vi "InclinometerSampleSensorLoop.vi"   [LabVIEW 2016]
uses:
  InclinometerSampleSensorLoopData.ctl
  InclinometerSampleSensorLoopStates.ctl
  InclinometerSample.ctl
  InclinometerErrorSample.ctl
  InclinometerErrorCodes.ctl
  <vilib>/Platform/TimedLoop/XDataNode/timing_clust.ctl
  <vilib>/Platform/TimedLoop/XDataNode/nitl_modes.ctl
  <vilib>/Platform/TimedLoop/XDataNode/wakeup.ctl
  <vilib>/rvi/Emulation/niFpgaSctlEmulationGetInTimedLoop.vi
  <vilib>/rvi/Emulation/niFpgaEmulationReportErrorSimple.vi
  <vilib>/rvi/Emulation/niFpgaGetClockAttributes.vi
  <vilib>/rvi/Emulation/niFpgaCriticalErrorInLSC.vi
  <vilib>/rvi/Emulation/niFpgaEmulationIsFPGAContextNoSignature.vi
  <vilib>/rvi/errors/niFpgaSetErrorForExecOnDevCompSimple.vi
  <vilib>/rvi/eio/common/nirviEmuReportErrorAndStop.vi
  <vilib>/rvi/DataTransferAndStorage/Container/Common/niFpgaContainerGetUniqueNameForEmu.vi
  <vilib>/rvi/FIFO/Fifo_Resource/nirvififoEmulationSetSize.vi
  <vilib>/rvi/FIFO/Fifo_Resource/nirviFifoEmulationQueueMgr.vi
  <instcachedir>/0/nirviFifoEmulationQueueMgr_E5CAEC123FF24DC58D834DCA3CDAA9B5.lvgen/nirviFifoEmulationQueueMgr_E5CAEC123FF24DC58D834DCA3CDAA9B5_004.vi
  <vilib>/Utility/error.llb/Clear Errors.vi
  <vilib>/rvi/FIFO/Fifo_Resource/nirvififoEmulationCreateLock.vi
  <vilib>/rvi/Emulation/niFpgaProcessEmulError.vi
  <vilib>/rvi/FIFO/Fifo_Resource/nirvififoEmulationObtainLock.vi
  <vilib>/rvi/FIFO/Fifo_Resource/nirvififoEmulationReleaseLock.vi
  <vilib>/rvi/occurrence/nirviWaitOnOccurrenceBase.vi
  <vilib>/rvi/errors/nirviReportUnexpectedCaseInternalError.vi
  <vilib>/rvi/errors/nirviReportUnexpectedCaseInternalError (U32).vi
  <vilib>/rvi/FIFO/Fifo_Resource/nirvififoEmulationDetermineInputValidOut.vi
  <instcachedir>/0/nirviFifoEmulationQueueMgr_E5CAEC123FF24DC58D834DCA3CDAA9B5.lvgen/nirviFifoEmulationQueueMgr_E5CAEC123FF24DC58D834DCA3CDAA9B5_009.vi
  <instcachedir>/0/nirviFifoEmulationQueueMgr_E5CAEC123FF24DC58D834DCA3CDAA9B5.lvgen/nirviFifoEmulationQueueMgr_E5CAEC123FF24DC58D834DCA3CDAA9B5_002.vi
  <vilib>/rvi/Memory/Memory_Emulation/niFpgaMemoryEmulationCacheClearOnFirstRun.vi
  <vilib>/rvi/Memory/Memory_Emulation/nirvimemoryEmulationManagerCache_MakeExclusive.vi
  <vilib>/rvi/Memory/Memory_Emulation/niFpgaMemoryEmulationValidateCache.vi
  <vilib>/rvi/Memory/Memory_Emulation/nirvimemoryEmulationManagerCache_InsertValue.vi
  <vilib>/rvi/Memory/Memory_Emulation/nirvimemoryEmulationManagerCache_ReleaseExclusive.vi
  <vilib>/rvi/Memory/Memory_Emulation/nirvimemoryEmulationManagerCache_GetValue.vi
  <vilib>/rvi/Memory/Memory_Emulation/nirvimemoryEmulationManagerCache_SetValue.vi
  <instcachedir>/0/nirviFifoEmulationQueueMgr_E5CAEC123FF24DC58D834DCA3CDAA9B5.lvgen/nirviFifoEmulationQueueMgr_E5CAEC123FF24DC58D834DCA3CDAA9B5_046.vi
  <instcachedir>/0/nirviFifoEmulationQueueMgr_E5CAEC123FF24DC58D834DCA3CDAA9B5.lvgen/nirviFifoEmulationQueueMgr_E5CAEC123FF24DC58D834DCA3CDAA9B5_033.vi
  <vilib>/Platform/TimedLoop/XDataNode/XDataNode.xnode
  <vilib>/rvi/DataTransferAndStorage/Container/XNode/niFpgaContainer.xnode
  <vilib>/rvi/FIFO/Fifo_Resource/nirvififoEmulationRead.vi
  <vilib>/rvi/FIFO/Fifo_Resource/nirvififoEmulationWrite.vi
  <vilib>/rvi/DataTransferAndStorage/Register/Emulation/niFpgaRegisterEmulation.vi
  <vilib>/Platform/TimedLoop/XDataNode/XDNodeRunTimeDep.lvlib
types:
  T1 = typedef "InclinometerSampleSensorLoopData.ctl" = cluster{"State":T2, "Timestamp":u64, "Timeout":i32, "Angle":u32, "CRC":u16, "Exception":u8, "Sample":T3, "ErrorSample":T4}
  T2 = typedef "InclinometerSampleSensorLoopStates.ctl" = enum16{"WaitForTrigger", "ClearRxFIFO", "WaitForClearComplete", "WriteAddress", "WriteFunction", "WriteStartAddress1", "WriteStartAddress0", "WriteAddressCount1", "WriteAddressCount0", "WriteCRC1", "WriteCRC0", "ReadAddress", "ReadFunction", "ReadByteCount", "ReadDataByte1", "ReadDataByte0", "ReadDataByte3", "ReadDataByte2", "ReadCRCByte0", "ReadCRCByte1", "CalculateCRC", "ValidateCRC", "PrepareSample", "MoveSample", "ReadExceptionCode", "ReadExceptionCRCByte0", "ReadExceptionCRCByte1", "CalculateExceptionCRC", "ValidateExceptionCRC", "ParseExceptionCode", "ResponseAddressError", "ResponseFunctionCodeError", "ResponseByteCountError", "ResponseCRCError", "ResponseUnknownError", "ResponseTimeoutError", "SensorReportsIllegalFunction", "SensorReportsIllegalDataAddress", "PrepareErrorCode", "MoveErrorCode"}
  T3 = typedef "InclinometerSample.ctl" = cluster{"Timestamp":u64, "TxBytes":u64, "RxBytes":u64, "TxFrames":u64, "RxFrames":u64, "RawAngle":i32}
  T4 = typedef "InclinometerErrorSample.ctl" = cluster{"Timestamp":u64, "TxBytes":u64, "RxBytes":u64, "TxFrames":u64, "RxFrames":u64, "ErrorCode":T5}
  T5 = typedef "InclinometerErrorCodes.ctl" = enum8{"None", "ResponseAddressError", "ResponseFunctionCodeError", "ResponseByteCountError", "ResponseCRCError", "ResponseUnknownError", "ResponseTimeoutError", "SensorReportsIllegalFunction", "SensorReportsIllegalDataAddress"}
  T6 = typedef "XDNodeRunTimeDep.lvlib/timing_clust.ctl" = cluster{"Expected End [f-1]":u64, "Actual End [f-1]":u64, "Finished Late? [f-1]":bool, "Expected End [i-1]":u64, "Actual End [i-1]":u64, "Finished Late? [i-1]":bool, "Expected Start [i]":u64, "Actual Start [i]":u64, "Expected Start [f]":u64, "Actual Start [f]":u64, "Source Name":string, "Structure Name":string, "Period":i64, "Deadline":i64, "Offset":i64, "Start":i64, "Priority":i32, "Timeout":i32, "Mode":T7, "Wakeup Reason":T8, "Error":errorcluster, "Source Type":string, "Secondary Source Type":string, "Global End Time":u64, "Global Start Time":u64, "Frame Duration":u64, "Iteration Duration":u64, "Assigned CPU":i32, "I/O Scan Engine Mode":u32}
  T7 = typedef "XDNodeRunTimeDep.lvlib/nitl_modes.ctl" = enum32{"No Change", "Process missed periods, maintain original phase", "Discard missed periods, maintain original phase", "Process missed periods, ignore original phase", "Discard missed periods, ignore original phase"}
  T8 = typedef "XDNodeRunTimeDep.lvlib/wakeup.ctl" = enum32{"Normal", "Aborted", "Asynchronous wakeup", "Timing source error", "Timed loop error", "Timeout"}
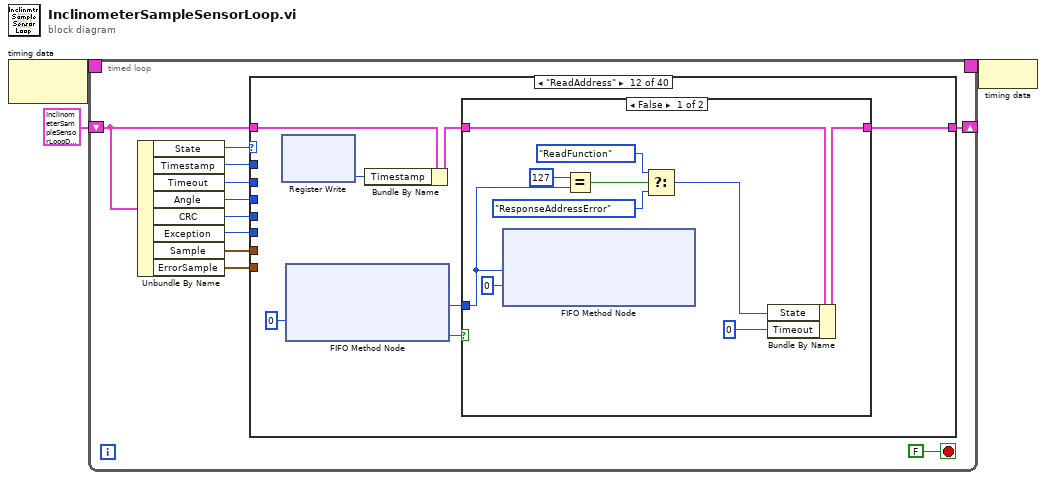
[diagram p0: block diagram]
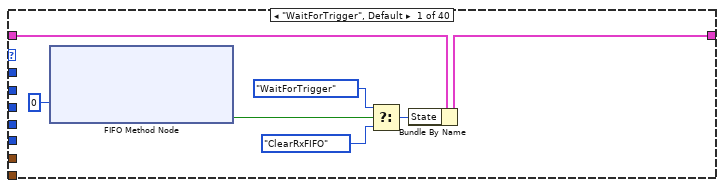
[diagram p2: hidden frame]
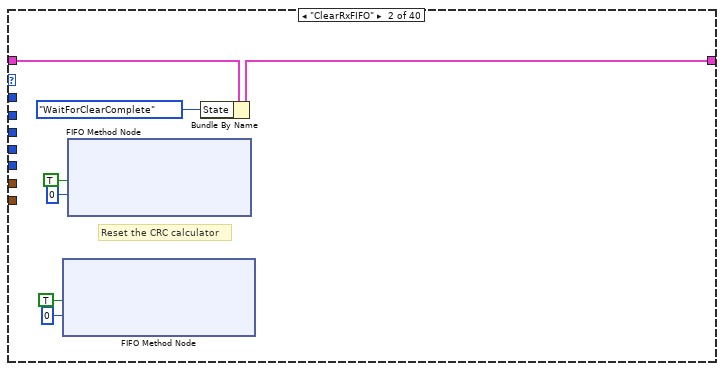
[diagram p3: hidden frame]
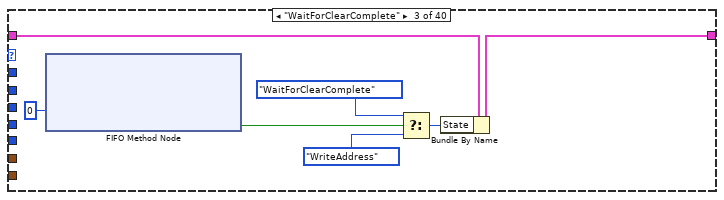
[diagram p4: hidden frame]
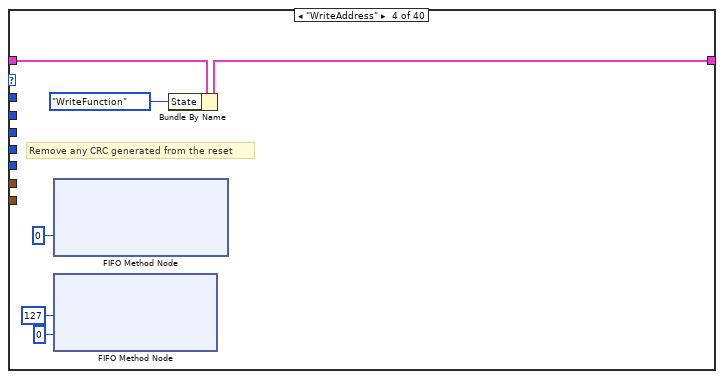
[diagram p5: hidden frame]
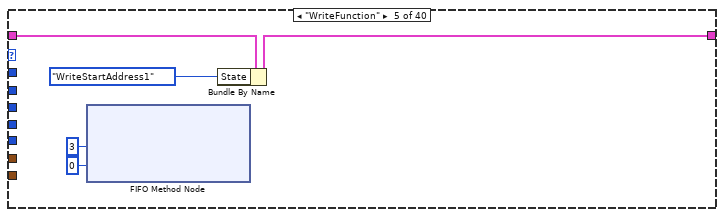
[diagram p6: hidden frame]
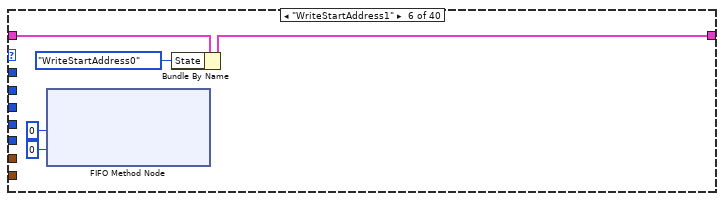
[diagram p7: hidden frame]
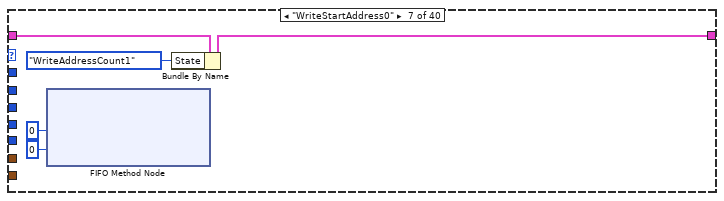
[diagram p8: hidden frame]
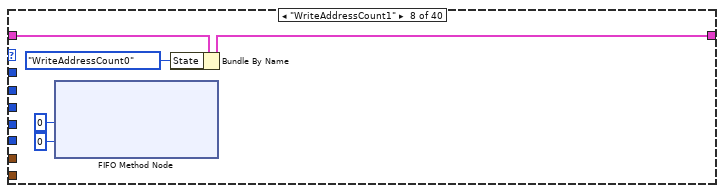
[diagram p9: hidden frame]
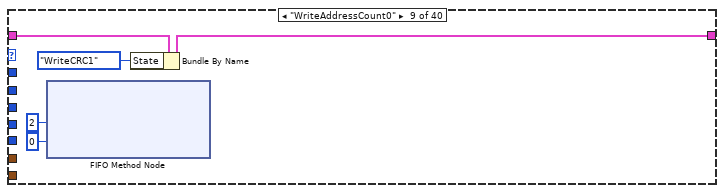
[diagram p10: hidden frame]
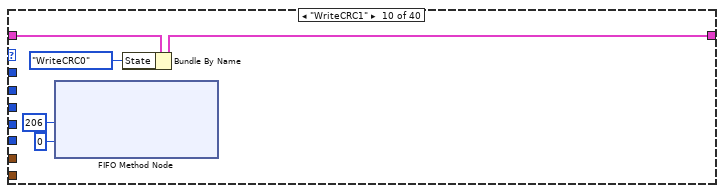
[diagram p11: hidden frame]
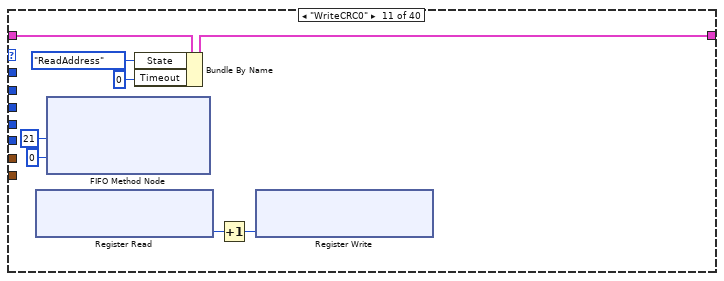
[diagram p12: hidden frame]
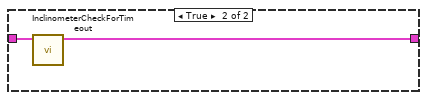
[diagram p13: hidden frame]
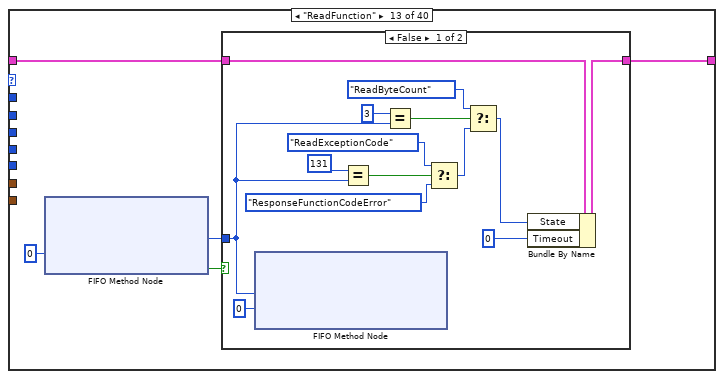
[diagram p14: hidden frame]
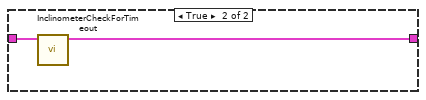
[diagram p15: hidden frame]
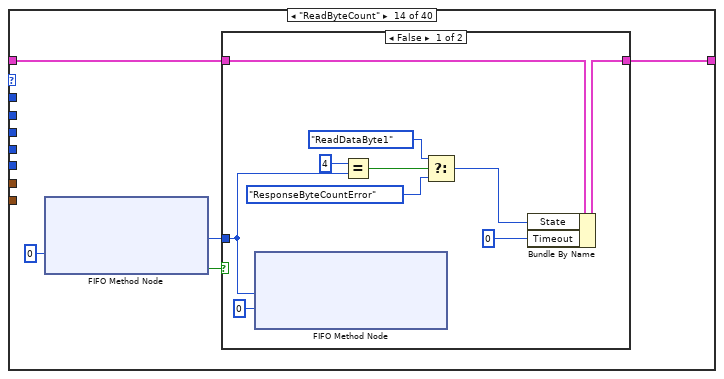
[diagram p16: hidden frame]
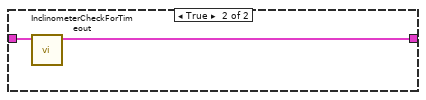
[diagram p17: hidden frame]
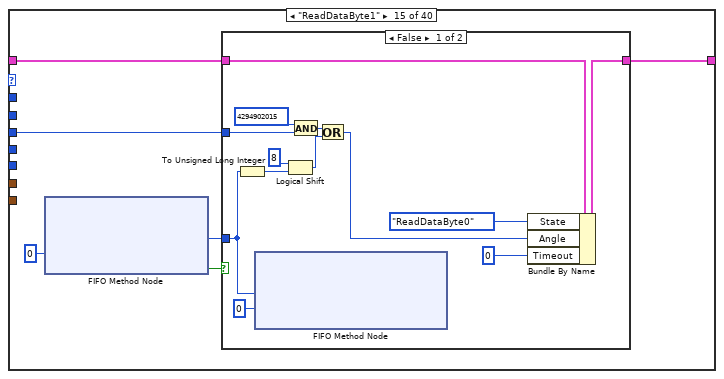
[diagram p18: hidden frame]
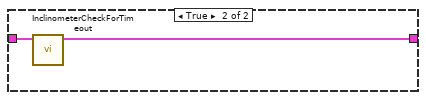
[diagram p19: hidden frame]
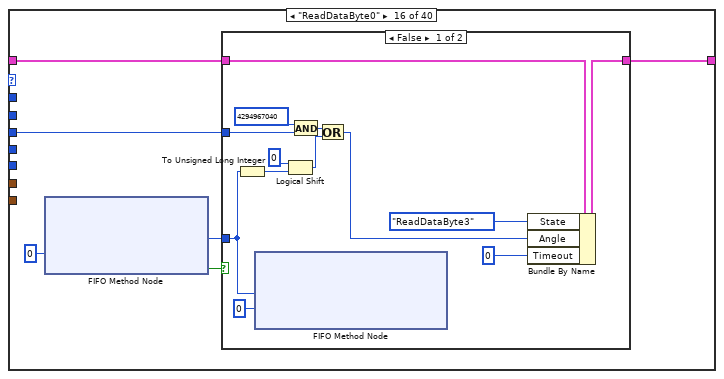
[diagram p20: hidden frame]
diagram:
  n1 = node-c288() -> (w3:T6)  [unwired: 1 in]
  n2 = timed-loop {
    timing: w3 -> [_]
    timing-out: [_] -> w2
    shift-right: [w13] -> _
    shift-left: T1 {"State"=enum."WaitForTrigger", "Timestamp"=0, "Timeout"=0, "Angle"=0, "CRC"=0, "Exception"=0, "Sample"={"Timestamp"=0, "TxBytes"=0, "RxBytes"=0, "TxFrames"=0, "RxFrames"=0, "RawAngle"=0}, "ErrorSample"={"Timestamp"=0, "TxBytes"=0, "RxBytes"=0, "TxFrames"=0, "RxFrames"=0, "ErrorCode"=enum."None"}} ("InclinometerData") -> [w14]
    stop <- FALSE stop-if-true
    n3 = Unbundle By Name(w14) -> ("State"=w12:T2, "Timestamp"=w7:u64, "Timeout"=w11:i32, "Angle"=w10:u32, "CRC"=w9:u16, "Exception"=w6:u8, "Sample"=w5:T3, "ErrorSample"=w4:T4)
    n4 = case shown="\"ReadAddress\"" w12 {
      tunnel: w14 -> [w20 w27 w34 w40 w45 w50 w55 w60 w65 w70 w78 w82 w99 w120 w138 w159 w180 w201 w222 w242 w264 w267 w290 w295 w297 w318 w338 w360 w363 w385 w389 w393 w397 w401 w405 w409 w413 w417 w425 w430]
      tunnel: [w21 w28 w35 w41 w46 w51 w56 w61 w66 w71 w79 w83 w100 w121 w139 w160 w181 w202 w223 w243 w265 w268 w291 w296 w298 w319 w339 w361 w364 w386 w390 w394 w398 w402 w406 w410 w414 w418 w426 w431] -> w13
      tunnel: w11 -> [_ _ _ _ _ _ _ _ _ _ _ _ _ _ _ _ _ _ _ _ _ _ _ _ _ _ _ _ _ _ _ _ _ _ _ _ _ _ _ _]
      tunnel: w10 -> [_ _ _ _ _ _ _ _ _ _ _ _ _ _ w137 w158 w179 w200 _ _ _ _ w284 _ _ _ _ _ _ _ _ _ _ _ _ _ _ _ _ _]
      tunnel: w9 -> [_ _ _ _ _ _ _ _ _ _ _ _ _ _ _ _ _ _ w221 w241 _ w266 _ _ _ w317 w337 _ w362 _ _ _ _ _ _ _ _ _ _ _]
      tunnel: w7 -> [_ _ _ _ _ _ _ _ _ _ _ _ _ _ _ _ _ _ _ _ _ _ w289 _ _ _ _ _ _ _ _ _ _ _ _ _ _ _ w424 _]
      tunnel: w6 -> [_ _ _ _ _ _ _ _ _ _ _ _ _ _ _ _ _ _ _ _ _ _ _ _ _ _ _ _ _ w380 _ _ _ _ _ _ _ _ _ _]
      tunnel: w5 -> [_ _ _ _ _ _ _ _ _ _ _ _ _ _ _ _ _ _ _ _ _ _ _ w294 _ _ _ _ _ _ _ _ _ _ _ _ _ _ _ _]
      tunnel: w4 -> [_ _ _ _ _ _ _ _ _ _ _ _ _ _ _ _ _ _ _ _ _ _ _ _ _ _ _ _ _ _ _ _ _ _ _ _ _ _ _ w427]
      frame "WaitForTrigger", Default {
        n5 = xnode ("FIFO Method Node")("Timeout"=0) -> ("Timed Out?"=w15:bool)  [unwired: 1 in, 2 out]
        n6 = Select(t=InclinometerSampleSensorLoopStates."WaitForTrigger" ("InclinometerState"), s=w15, f=InclinometerSampleSensorLoopStates."ClearRxFIFO" ("InclinometerState")) -> (s? t:f=w17:T2)
        n7 = Bundle By Name(cluster=w20, "State"=w17) -> (w21:T1)
      }
      frame "ClearRxFIFO" {
        # "Reset the CRC calculator"
        n8 = xnode ("FIFO Method Node")("Element"=TRUE, "Timeout"=0) -> ()  [unwired: 1 in, 2 out]
        n9 = xnode ("FIFO Method Node")("Element"=TRUE, "Timeout"=0) -> ()  [unwired: 1 in, 2 out]
        n10 = Bundle By Name(cluster=w27, "State"=InclinometerSampleSensorLoopStates."WaitForClearComplete" ("InclinometerState")) -> (w28:T1)
      }
      frame "WaitForClearComplete" {
        n11 = xnode ("FIFO Method Node")("Timeout"=0) -> ("Timed Out?"=w29:bool)  [unwired: 1 in, 2 out]
        n12 = Select(t=InclinometerSampleSensorLoopStates."WaitForClearComplete", s=w29, f=InclinometerSampleSensorLoopStates."WriteAddress" ("InclinometerState")) -> (s? t:f=w31:T2)
        n13 = Bundle By Name(cluster=w34, "State"=w31) -> (w35:T1)
      }
      frame "WriteAddress" {
        # "Remove any CRC generated from the reset"
        n14 = xnode ("FIFO Method Node")("Timeout"=0) -> ()  [unwired: 1 in, 3 out]
        n15 = xnode ("FIFO Method Node")("Element"=u8 127, "Timeout"=0) -> ()  [unwired: 1 in, 2 out]
        n16 = Bundle By Name(cluster=w40, "State"=InclinometerSampleSensorLoopStates."WriteFunction" ("InclinometerState")) -> (w41:T1)
      }
      frame "WriteFunction" {
        n17 = xnode ("FIFO Method Node")("Element"=u8 3, "Timeout"=0) -> ()  [unwired: 1 in, 2 out]
        n18 = Bundle By Name(cluster=w45, "State"=InclinometerSampleSensorLoopStates."WriteStartAddress1" ("InclinometerState")) -> (w46:T1)
      }
      frame "WriteStartAddress1" {
        n19 = xnode ("FIFO Method Node")("Element"=u8 0, "Timeout"=0) -> ()  [unwired: 1 in, 2 out]
        n20 = Bundle By Name(cluster=w50, "State"=InclinometerSampleSensorLoopStates."WriteStartAddress0" ("InclinometerState")) -> (w51:T1)
      }
      frame "WriteStartAddress0" {
        n21 = xnode ("FIFO Method Node")("Element"=u8 0, "Timeout"=0) -> ()  [unwired: 1 in, 2 out]
        n22 = Bundle By Name(cluster=w55, "State"=InclinometerSampleSensorLoopStates."WriteAddressCount1" ("InclinometerState")) -> (w56:T1)
      }
      frame "WriteAddressCount1" {
        n23 = xnode ("FIFO Method Node")("Element"=u8 0, "Timeout"=0) -> ()  [unwired: 1 in, 2 out]
        n24 = Bundle By Name(cluster=w60, "State"=InclinometerSampleSensorLoopStates."WriteAddressCount0" ("InclinometerState")) -> (w61:T1)
      }
      frame "WriteAddressCount0" {
        n25 = xnode ("FIFO Method Node")("Element"=u8 2, "Timeout"=0) -> ()  [unwired: 1 in, 2 out]
        n26 = Bundle By Name(cluster=w65, "State"=InclinometerSampleSensorLoopStates."WriteCRC1" ("InclinometerState")) -> (w66:T1)
      }
      frame "WriteCRC1" {
        n27 = xnode ("FIFO Method Node")("Element"=u8 206, "Timeout"=0) -> ()  [unwired: 1 in, 2 out]
        n28 = Bundle By Name(cluster=w70, "State"=InclinometerSampleSensorLoopStates."WriteCRC0" ("InclinometerState")) -> (w71:T1)
      }
      frame "WriteCRC0" {
        n29 = xnode ("Register Read")() -> ("Data"=w73:u64)  [unwired: 1 in, 1 out]
        n30 = xnode ("FIFO Method Node")("Element"=u8 21, "Timeout"=0) -> ()  [unwired: 1 in, 2 out]
        n31 = Bundle By Name(cluster=w78, "State"=InclinometerSampleSensorLoopStates."ReadAddress" ("InclinometerState"), "Timeout"=0) -> (w79:T1)
        n32 = Increment(x=w73) -> (x+1=w72:u64)
        n33 = xnode ("Register Write")("Data"=w72) -> ()  [unwired: 1 in, 1 out]
      }
      frame "ReadAddress" {
        n34 = xnode "Register Write"() -> ("Data"=w80:u64)  [unwired: 1 in, 1 out]
        n35 = xnode ("FIFO Method Node")("Timeout"=0) -> ("Element"=w84:u8, "Timed Out?"=w85:bool)  [unwired: 1 in, 1 out]
        n36 = Bundle By Name(cluster=w82, "Timestamp"=w80) -> (w81:T1)
        n37 = case shown="False" w85 {
          tunnel: w84 -> [w93 _]
          tunnel: [w95 w97] -> w83
          tunnel: w81 -> [w96 w98]
          frame False {
            n38 = xnode ("FIFO Method Node")("Element"=w93, "Timeout"=0) -> ()  [unwired: 1 in, 2 out]
            n39 = Equal?(x=u8 127, y=w93) -> (x = y?=w91:bool)
            n40 = Select(t=InclinometerSampleSensorLoopStates."ReadFunction" ("InclinometerState"), s=w91, f=InclinometerSampleSensorLoopStates."ResponseAddressError" ("InclinometerState")) -> (s? t:f=w88:T2)
            n41 = Bundle By Name(cluster=w96, "State"=w88, "Timeout"=0) -> (w95:T1)
          }
          frame True {
            n42 = call "InclinometerCheckForTimeout.vi"("InclinometerSampleSensorLoopData in"=w98) -> ("InclinometerSampleSensorLoopData out"=w97:T1)  [unwired: 10 in]
          }
        }
      }
      frame "ReadFunction" {
        n43 = xnode ("FIFO Method Node")("Timeout"=0) -> ("Element"=w101:u8, "Timed Out?"=w102:bool)  [unwired: 1 in, 1 out]
        n44 = case shown="False" w102 {
          tunnel: w101 -> [w109 _]
          tunnel: [w116 w118] -> w100
          tunnel: w99 -> [w117 w119]
          frame False {
            n45 = xnode ("FIFO Method Node")("Element"=w109, "Timeout"=0) -> ()  [unwired: 1 in, 2 out]
            n46 = Equal?(x=u8 131, y=w109) -> (x = y?=w108:bool)
            n47 = Equal?(x=u8 3, y=w109) -> (x = y?=w113:bool)
            n48 = Select(t=InclinometerSampleSensorLoopStates."ReadExceptionCode" ("InclinometerState"), s=w108, f=InclinometerSampleSensorLoopStates."ResponseFunctionCodeError" ("InclinometerState")) -> (s? t:f=w111:T2)
            n49 = Select(t=InclinometerSampleSensorLoopStates."ReadByteCount" ("InclinometerState"), s=w113, f=w111) -> (s? t:f=w105:T2)
            n50 = Bundle By Name(cluster=w117, "State"=w105, "Timeout"=0) -> (w116:T1)
          }
          frame True {
            n51 = call "InclinometerCheckForTimeout.vi"("InclinometerSampleSensorLoopData in"=w119) -> ("InclinometerSampleSensorLoopData out"=w118:T1)  [unwired: 10 in]
          }
        }
      }
      frame "ReadByteCount" {
        n52 = xnode ("FIFO Method Node")("Timeout"=0) -> ("Element"=w122:u8, "Timed Out?"=w123:bool)  [unwired: 1 in, 1 out]
        n53 = case shown="False" w123 {
          tunnel: w122 -> [w131 _]
          tunnel: [w133 w135] -> w121
          tunnel: w120 -> [w134 w136]
          frame False {
            n54 = xnode ("FIFO Method Node")("Element"=w131, "Timeout"=0) -> ()  [unwired: 1 in, 2 out]
            n55 = Equal?(x=u8 4, y=w131) -> (x = y?=w129:bool)
            n56 = Select(t=InclinometerSampleSensorLoopStates."ReadDataByte1" ("InclinometerState"), s=w129, f=InclinometerSampleSensorLoopStates."ResponseByteCountError" ("InclinometerState")) -> (s? t:f=w126:T2)
            n57 = Bundle By Name(cluster=w134, "State"=w126, "Timeout"=0) -> (w133:T1)
          }
          frame True {
            n58 = call "InclinometerCheckForTimeout.vi"("InclinometerSampleSensorLoopData in"=w136) -> ("InclinometerSampleSensorLoopData out"=w135:T1)  [unwired: 10 in]
          }
        }
      }
      frame "ReadDataByte1" {
        n59 = xnode ("FIFO Method Node")("Timeout"=0) -> ("Element"=w140:u8, "Timed Out?"=w141:bool)  [unwired: 1 in, 1 out]
        n60 = case shown="False" w141 {
          tunnel: w140 -> [w146 _]
          tunnel: [w154 w156] -> w139
          tunnel: w138 -> [w155 w157]
          tunnel: w137 -> [w150 _]
          frame False {
            n61 = To Unsigned Long Integer(number=w146) -> (unsigned 32bit integer=w145:u32)
            n62 = xnode ("FIFO Method Node")("Element"=w146, "Timeout"=0) -> ()  [unwired: 1 in, 2 out]
            n63 = Logical Shift(y=i16 8, x=w145) -> (x << y=w148:u32)
            n64 = And(x=u32 4294902015, y=w150) -> (x .and. y?=w147:u32)
            n65 = Or(x=w147, y=w148) -> (x .or. y?=w144:u32)
            n66 = Bundle By Name(cluster=w155, "State"=InclinometerSampleSensorLoopStates."ReadDataByte0" ("InclinometerState"), "Angle"=w144, "Timeout"=0) -> (w154:T1)
          }
          frame True {
            n67 = call "InclinometerCheckForTimeout.vi"("InclinometerSampleSensorLoopData in"=w157) -> ("InclinometerSampleSensorLoopData out"=w156:T1)  [unwired: 10 in]
          }
        }
      }
      frame "ReadDataByte0" {
        n68 = xnode ("FIFO Method Node")("Timeout"=0) -> ("Element"=w161:u8, "Timed Out?"=w162:bool)  [unwired: 1 in, 1 out]
        n69 = case shown="False" w162 {
          tunnel: w161 -> [w167 _]
          tunnel: [w175 w177] -> w160
          tunnel: w159 -> [w176 w178]
          tunnel: w158 -> [w171 _]
          frame False {
            n70 = To Unsigned Long Integer(number=w167) -> (unsigned 32bit integer=w166:u32)
            n71 = xnode ("FIFO Method Node")("Element"=w167, "Timeout"=0) -> ()  [unwired: 1 in, 2 out]
            n72 = Logical Shift(y=i16 0, x=w166) -> (x << y=w169:u32)
            n73 = And(x=u32 4294967040, y=w171) -> (x .and. y?=w168:u32)
            n74 = Or(x=w168, y=w169) -> (x .or. y?=w165:u32)
            n75 = Bundle By Name(cluster=w176, "State"=InclinometerSampleSensorLoopStates."ReadDataByte3" ("InclinometerState"), "Angle"=w165, "Timeout"=0) -> (w175:T1)
          }
          frame True {
            n76 = call "InclinometerCheckForTimeout.vi"("InclinometerSampleSensorLoopData in"=w178) -> ("InclinometerSampleSensorLoopData out"=w177:T1)  [unwired: 10 in]
          }
        }
      }
      frame "ReadDataByte3" {
        n77 = xnode ("FIFO Method Node")("Timeout"=0) -> ("Element"=w182:u8, "Timed Out?"=w183:bool)  [unwired: 1 in, 1 out]
        n78 = case shown="False" w183 {
          tunnel: w182 -> [w188 _]
          tunnel: [w196 w198] -> w181
          tunnel: w180 -> [w197 w199]
          tunnel: w179 -> [w192 _]
          frame False {
            n79 = To Unsigned Long Integer(number=w188) -> (unsigned 32bit integer=w187:u32)
            n80 = xnode ("FIFO Method Node")("Element"=w188, "Timeout"=0) -> ()  [unwired: 1 in, 2 out]
            n81 = Logical Shift(y=i16 24, x=w187) -> (x << y=w190:u32)
            n82 = And(x=u32 16777215, y=w192) -> (x .and. y?=w189:u32)
            n83 = Or(x=w189, y=w190) -> (x .or. y?=w186:u32)
            n84 = Bundle By Name(cluster=w197, "State"=InclinometerSampleSensorLoopStates."ReadDataByte2" ("InclinometerState"), "Angle"=w186, "Timeout"=0) -> (w196:T1)
          }
          frame True {
            n85 = call "InclinometerCheckForTimeout.vi"("InclinometerSampleSensorLoopData in"=w199) -> ("InclinometerSampleSensorLoopData out"=w198:T1)  [unwired: 10 in]
          }
        }
      }
      frame "ReadDataByte2" {
        n86 = xnode ("FIFO Method Node")("Timeout"=0) -> ("Element"=w203:u8, "Timed Out?"=w204:bool)  [unwired: 1 in, 1 out]
        n87 = case shown="False" w204 {
          tunnel: w203 -> [w209 _]
          tunnel: [w217 w219] -> w202
          tunnel: w201 -> [w218 w220]
          tunnel: w200 -> [w213 _]
          frame False {
            n88 = To Unsigned Long Integer(number=w209) -> (unsigned 32bit integer=w208:u32)
            n89 = xnode ("FIFO Method Node")("Element"=w209, "Timeout"=0) -> ()  [unwired: 1 in, 2 out]
            n90 = Logical Shift(y=i16 16, x=w208) -> (x << y=w211:u32)
            n91 = And(x=u32 4278255615, y=w213) -> (x .and. y?=w210:u32)
            n92 = Or(x=w210, y=w211) -> (x .or. y?=w207:u32)
            n93 = Bundle By Name(cluster=w218, "State"=InclinometerSampleSensorLoopStates."ReadCRCByte0" ("InclinometerState"), "Angle"=w207, "Timeout"=0) -> (w217:T1)
          }
          frame True {
            n94 = call "InclinometerCheckForTimeout.vi"("InclinometerSampleSensorLoopData in"=w220) -> ("InclinometerSampleSensorLoopData out"=w219:T1)  [unwired: 10 in]
          }
        }
      }
      frame "ReadCRCByte0" {
        n95 = xnode ("FIFO Method Node")("Timeout"=0) -> ("Element"=w224:u8, "Timed Out?"=w225:bool)  [unwired: 1 in, 1 out]
        n96 = case shown="False" w225 {
          tunnel: w224 -> [w231 _]
          tunnel: [w237 w239] -> w223
          tunnel: w222 -> [w238 w240]
          tunnel: w221 -> [w228 _]
          frame False {
            n97 = To Unsigned Word Integer(number=w231) -> (unsigned 16bit integer=w230:u16)
            n98 = Logical Shift(y=i16 0, x=w230) -> (x << y=w233:u16)
            n99 = And(x=u16 65280, y=w228) -> (x .and. y?=w232:u16)
            n100 = Or(x=w232, y=w233) -> (x .or. y?=w229:u16)
            n101 = Bundle By Name(cluster=w238, "State"=InclinometerSampleSensorLoopStates."ReadCRCByte1" ("InclinometerState"), "CRC"=w229, "Timeout"=0) -> (w237:T1)
          }
          frame True {
            n102 = call "InclinometerCheckForTimeout.vi"("InclinometerSampleSensorLoopData in"=w240) -> ("InclinometerSampleSensorLoopData out"=w239:T1)  [unwired: 10 in]
          }
        }
      }
      frame "ReadCRCByte1" {
        n103 = xnode ("FIFO Method Node")("Timeout"=0) -> ("Element"=w244:u8, "Timed Out?"=w245:bool)  [unwired: 1 in, 1 out]
        n104 = case shown="False" w245 {
          tunnel: w244 -> [w251 _]
          tunnel: [w257 w259] -> w243
          tunnel: w242 -> [w258 w260]
          tunnel: w241 -> [w248 _]
          frame False {
            n105 = To Unsigned Word Integer(number=w251) -> (unsigned 16bit integer=w250:u16)
            n106 = Logical Shift(y=i16 8, x=w250) -> (x << y=w253:u16)
            n107 = And(x=u16 255, y=w248) -> (x .and. y?=w252:u16)
            n108 = Or(x=w252, y=w253) -> (x .or. y?=w249:u16)
            n109 = Bundle By Name(cluster=w258, "State"=InclinometerSampleSensorLoopStates."CalculateCRC" ("InclinometerState"), "CRC"=w249, "Timeout"=0) -> (w257:T1)
          }
          frame True {
            n110 = call "InclinometerCheckForTimeout.vi"("InclinometerSampleSensorLoopData in"=w260) -> ("InclinometerSampleSensorLoopData out"=w259:T1)  [unwired: 10 in]
          }
        }
      }
      frame "CalculateCRC" {
        n111 = xnode ("FIFO Method Node")("Element"=TRUE, "Timeout"=0) -> ()  [unwired: 1 in, 2 out]
        n112 = Bundle By Name(cluster=w264, "State"=InclinometerSampleSensorLoopStates."ValidateCRC" ("InclinometerState")) -> (w265:T1)
      }
      frame "ValidateCRC" {
        n113 = xnode ("FIFO Method Node")("Timeout"=0) -> ("Element"=w269:u16, "Timed Out?"=w270:bool)  [unwired: 1 in, 1 out]
        n114 = case shown="False" w270 {
          tunnel: w269 -> [w274 _]
          tunnel: [w280 w282] -> w268
          tunnel: w267 -> [w281 w282]
          tunnel: w266 -> [w275 _]
          frame False {
            n115 = xnode ("Register Read")() -> ("Data"=w272:u64)  [unwired: 1 in, 1 out]
            n116 = Equal?(x=w275, y=w274) -> (x = y?=w279:bool)
            n117 = Select(t=InclinometerSampleSensorLoopStates."PrepareSample" ("InclinometerState"), s=w279, f=InclinometerSampleSensorLoopStates."ResponseCRCError" ("InclinometerState")) -> (s? t:f=w276:T2)
            n118 = Increment(x=w272) -> (x+1=w273:u64)
            n119 = xnode ("Register Write")("Data"=w273) -> ()  [unwired: 1 in, 1 out]
            n120 = Bundle By Name(cluster=w281, "State"=w276) -> (w280:T1)
          }
          frame True {
          }
        }
      }
      frame "PrepareSample" {
        n121 = xnode ("Register Read")() -> ("Data"=w288:u64)  [unwired: 1 in, 1 out]
        n122 = xnode ("Register Read")() -> ("Data"=w287:u64)  [unwired: 1 in, 1 out]
        n123 = xnode ("Register Read")() -> ("Data"=w286:u64)  [unwired: 1 in, 1 out]
        n124 = xnode ("Register Read")() -> ("Data"=w285:u64)  [unwired: 1 in, 1 out]
        n125 = Bundle By Name(cluster=w290, "State"=InclinometerSampleSensorLoopStates."MoveSample", "Sample.Timestamp"=w289, "Sample.TxBytes"=w288, "Sample.RxBytes"=w287, "Sample.TxFrames"=w286, "Sample.RxFrames"=w285, "Sample.RawAngle"=w284) -> (w291:T1)
      }
      frame "MoveSample" {
        n126 = xnode ("FIFO Method Node")("Element"=w294, "Timeout"=0) -> ()  [unwired: 1 in, 2 out]
        n127 = Bundle By Name(cluster=w295, "State"=InclinometerSampleSensorLoopStates."WaitForTrigger") -> (w296:T1)
      }
      frame "ReadExceptionCode" {
        n128 = xnode ("FIFO Method Node")("Timeout"=0) -> ("Element"=w299:u8, "Timed Out?"=w300:bool)  [unwired: 1 in, 1 out]
        n129 = case shown="False" w300 {
          tunnel: w299 -> [w302 _]
          tunnel: [w313 w315] -> w298
          tunnel: w297 -> [w314 w316]
          frame False {
            n130 = xnode ("FIFO Method Node")("Element"=w302, "Timeout"=0) -> ()  [unwired: 1 in, 2 out]
            n131 = Equal?(x=u8 1, y=w302) -> (x = y?=w305:bool)
            n132 = Equal?(x=u8 2, y=w302) -> (x = y?=w304:bool)
            n133 = Or(x=w305, y=w304) -> (x .or. y?=w303:bool)
            n134 = Select(t=InclinometerSampleSensorLoopStates."ReadExceptionCRCByte0" ("InclinometerState"), s=w303, f=InclinometerSampleSensorLoopStates."ResponseUnknownError" ("InclinometerState")) -> (s? t:f=w308:T2)
            n135 = Bundle By Name(cluster=w314, "State"=w308, "Timeout"=0, "Exception"=w302) -> (w313:T1)
          }
          frame True {
            n136 = call "InclinometerCheckForTimeout.vi"("InclinometerSampleSensorLoopData in"=w316) -> ("InclinometerSampleSensorLoopData out"=w315:T1)  [unwired: 10 in]
          }
        }
      }
      frame "ReadExceptionCRCByte0" {
        n137 = xnode ("FIFO Method Node")("Timeout"=0) -> ("Element"=w320:u8, "Timed Out?"=w321:bool)  [unwired: 1 in, 1 out]
        n138 = case shown="False" w321 {
          tunnel: w320 -> [w327 _]
          tunnel: [w333 w335] -> w319
          tunnel: w318 -> [w334 w336]
          tunnel: w317 -> [w324 _]
          frame False {
            n139 = To Unsigned Word Integer(number=w327) -> (unsigned 16bit integer=w326:u16)
            n140 = Logical Shift(y=i16 0, x=w326) -> (x << y=w329:u16)
            n141 = And(x=u16 65280, y=w324) -> (x .and. y?=w328:u16)
            n142 = Or(x=w328, y=w329) -> (x .or. y?=w325:u16)
            n143 = Bundle By Name(cluster=w334, "State"=InclinometerSampleSensorLoopStates."ReadExceptionCRCByte1" ("InclinometerState"), "CRC"=w325, "Timeout"=0) -> (w333:T1)
          }
          frame True {
            n144 = call "InclinometerCheckForTimeout.vi"("InclinometerSampleSensorLoopData in"=w336) -> ("InclinometerSampleSensorLoopData out"=w335:T1)  [unwired: 10 in]
          }
        }
      }
      frame "ReadExceptionCRCByte1" {
        n145 = xnode ("FIFO Method Node")("Timeout"=0) -> ("Element"=w340:u8, "Timed Out?"=w341:bool)  [unwired: 1 in, 1 out]
        n146 = case shown="False" w341 {
          tunnel: w340 -> [w347 _]
          tunnel: [w353 w355] -> w339
          tunnel: w338 -> [w354 w356]
          tunnel: w337 -> [w344 _]
          frame False {
            n147 = To Unsigned Word Integer(number=w347) -> (unsigned 16bit integer=w346:u16)
            n148 = Logical Shift(y=i16 8, x=w346) -> (x << y=w349:u16)
            n149 = And(x=u16 255, y=w344) -> (x .and. y?=w348:u16)
            n150 = Or(x=w348, y=w349) -> (x .or. y?=w345:u16)
            n151 = Bundle By Name(cluster=w354, "State"=InclinometerSampleSensorLoopStates."CalculateExceptionCRC" ("InclinometerState"), "CRC"=w345, "Timeout"=0) -> (w353:T1)
          }
          frame True {
            n152 = call "InclinometerCheckForTimeout.vi"("InclinometerSampleSensorLoopData in"=w356) -> ("InclinometerSampleSensorLoopData out"=w355:T1)  [unwired: 10 in]
          }
        }
      }
      frame "CalculateExceptionCRC" {
        n153 = xnode ("FIFO Method Node")("Element"=TRUE, "Timeout"=0) -> ()  [unwired: 1 in, 2 out]
        n154 = Bundle By Name(cluster=w360, "State"=InclinometerSampleSensorLoopStates."ValidateExceptionCRC" ("InclinometerState")) -> (w361:T1)
      }
      frame "ValidateExceptionCRC" {
        n155 = xnode ("FIFO Method Node")("Timeout"=0) -> ("Element"=w365:u16, "Timed Out?"=w366:bool)  [unwired: 1 in, 1 out]
        n156 = case shown="False" w366 {
          tunnel: w365 -> [w370 _]
          tunnel: [w376 w378] -> w364
          tunnel: w363 -> [w377 w378]
          tunnel: w362 -> [w371 _]
          frame False {
            n157 = xnode ("Register Read")() -> ("Data"=w369:u64)  [unwired: 1 in, 1 out]
            n158 = Equal?(x=w371, y=w370) -> (x = y?=w375:bool)
            n159 = Select(t=InclinometerSampleSensorLoopStates."ParseExceptionCode" ("InclinometerState"), s=w375, f=InclinometerSampleSensorLoopStates."ResponseCRCError" ("InclinometerState")) -> (s? t:f=w372:T2)
            n160 = Increment(x=w369) -> (x+1=w368:u64)
            n161 = xnode ("Register Write")("Data"=w368) -> ()  [unwired: 1 in, 1 out]
            n162 = Bundle By Name(cluster=w377, "State"=w372) -> (w376:T1)
          }
          frame True {
          }
        }
      }
      frame "ParseExceptionCode" {
        n163 = Equal?(x=w380, y=u8 1) -> (x = y?=w384:bool)
        n164 = Select(t=InclinometerSampleSensorLoopStates."SensorReportsIllegalFunction" ("InclinometerState"), s=w384, f=InclinometerSampleSensorLoopStates."SensorReportsIllegalDataAddress" ("InclinometerState")) -> (s? t:f=w381:T2)
        n165 = Bundle By Name(cluster=w385, "State"=w381) -> (w386:T1)
      }
      frame "ResponseAddressError" {
        n166 = Bundle By Name(cluster=w389, "State"=InclinometerSampleSensorLoopStates."PrepareErrorCode" ("InclinometerState"), "ErrorSample.ErrorCode"=InclinometerErrorCodes."ResponseAddressError" ("InclinometerErrorCodes")) -> (w390:T1)
      }
      frame "ResponseFunctionCodeError" {
        n167 = Bundle By Name(cluster=w393, "State"=InclinometerSampleSensorLoopStates."PrepareErrorCode" ("InclinometerState"), "ErrorSample.ErrorCode"=InclinometerErrorCodes."ResponseFunctionCodeError" ("InclinometerErrorCodes")) -> (w394:T1)
      }
      frame "ResponseByteCountError" {
        n168 = Bundle By Name(cluster=w397, "State"=InclinometerSampleSensorLoopStates."PrepareErrorCode" ("InclinometerState"), "ErrorSample.ErrorCode"=InclinometerErrorCodes."ResponseByteCountError" ("InclinometerErrorCodes")) -> (w398:T1)
      }
      frame "ResponseCRCError" {
        n169 = Bundle By Name(cluster=w401, "State"=InclinometerSampleSensorLoopStates."PrepareErrorCode" ("InclinometerState"), "ErrorSample.ErrorCode"=InclinometerErrorCodes."ResponseCRCError" ("InclinometerErrorCodes")) -> (w402:T1)
      }
      frame "ResponseUnknownError" {
        n170 = Bundle By Name(cluster=w405, "State"=InclinometerSampleSensorLoopStates."PrepareErrorCode" ("InclinometerState"), "ErrorSample.ErrorCode"=InclinometerErrorCodes."ResponseUnknownError" ("InclinometerErrorCodes")) -> (w406:T1)
      }
      frame "ResponseTimeoutError" {
        n171 = Bundle By Name(cluster=w409, "State"=InclinometerSampleSensorLoopStates."PrepareErrorCode" ("InclinometerState"), "ErrorSample.ErrorCode"=InclinometerErrorCodes."ResponseTimeoutError" ("InclinometerErrorCodes")) -> (w410:T1)
      }
      frame "SensorReportsIllegalFunction" {
        n172 = Bundle By Name(cluster=w413, "State"=InclinometerSampleSensorLoopStates."PrepareErrorCode" ("InclinometerState"), "ErrorSample.ErrorCode"=InclinometerErrorCodes."SensorReportsIllegalFunction" ("InclinometerErrorCodes")) -> (w414:T1)
      }
      frame "SensorReportsIllegalDataAddress" {
        n173 = Bundle By Name(cluster=w417, "State"=InclinometerSampleSensorLoopStates."PrepareErrorCode" ("InclinometerState"), "ErrorSample.ErrorCode"=InclinometerErrorCodes."SensorReportsIllegalDataAddress" ("InclinometerErrorCodes")) -> (w418:T1)
      }
      frame "PrepareErrorCode" {
        n174 = xnode ("Register Read")() -> ("Data"=w423:u64)  [unwired: 1 in, 1 out]
        n175 = xnode ("Register Read")() -> ("Data"=w422:u64)  [unwired: 1 in, 1 out]
        n176 = xnode ("Register Read")() -> ("Data"=w421:u64)  [unwired: 1 in, 1 out]
        n177 = xnode ("Register Read")() -> ("Data"=w420:u64)  [unwired: 1 in, 1 out]
        n178 = Bundle By Name(cluster=w425, "State"=InclinometerSampleSensorLoopStates."MoveErrorCode", "ErrorSample.Timestamp"=w424, "ErrorSample.TxBytes"=w423, "ErrorSample.RxBytes"=w422, "ErrorSample.TxFrames"=w421, "ErrorSample.RxFrames"=w420) -> (w426:T1)
      }
      frame "MoveErrorCode" {
        n179 = xnode ("FIFO Method Node")("Element"=w427, "Timeout"=0) -> ()  [unwired: 1 in, 2 out]
        n180 = Bundle By Name(cluster=w430, "State"=InclinometerSampleSensorLoopStates."WaitForTrigger") -> (w431:T1)
      }
    }
  }
  n181 = node-c288(w2) -> ()
